vi "extract data to circle.vi"(5 "Circles (Shape Detection 1)":T1(array[cluster]) {"Position"."Y" format="%.2f"; "Position"."X" format="%.2f"}) -> (0 "Circles":cluster{"x":dbl, "y":dbl, "r":dbl}[](array[cluster]), 1 "y":dbl[](array[numeric]), 2 "x":dbl[](array[numeric]))   [LabVIEW 2018]
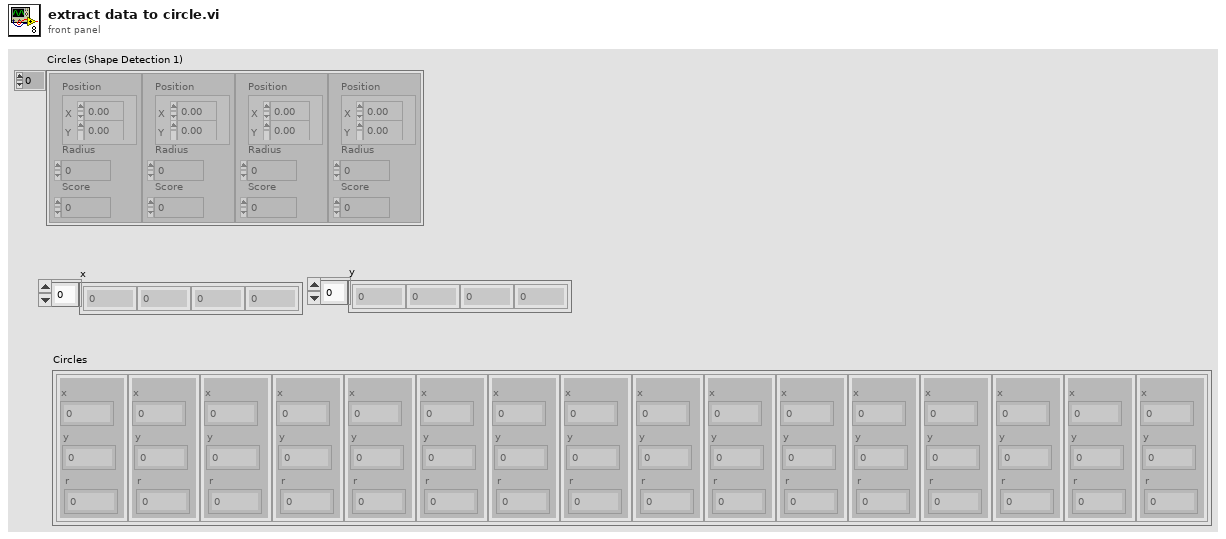
[diagram p1: front panel]
types:
  T1 = cluster{"Position":cluster{"X":sgl, "Y":sgl}, "Radius":dbl, "Score":dbl}[]
  T2 = cluster{"element":dbl, "element":dbl, "element":dbl}
  T3 = cluster{"element":dbl, "element":dbl, "element":dbl}[]
  T4 = cluster{"Position":cluster{"X":sgl, "Y":sgl}, "Radius":dbl, "Score":dbl}
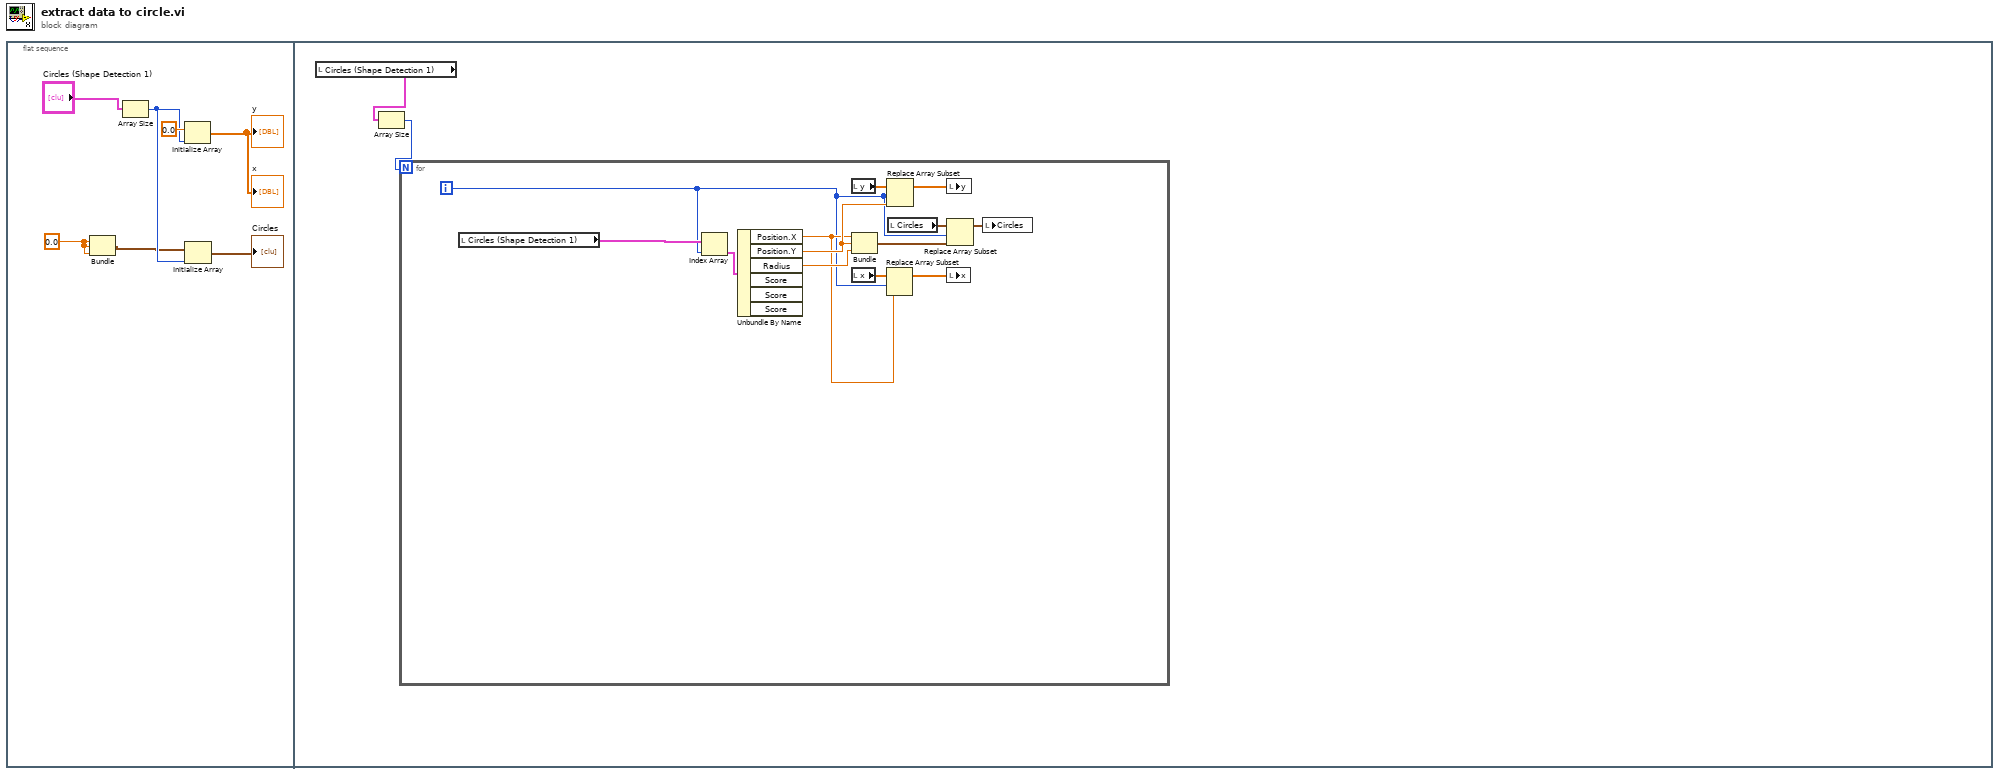
[diagram p0: block diagram]
diagram:
  n1 = flat-sequence {
    frame #0 {
      w1 = 0.0 ("element")
      n2 = Bundle("element"=w1, "element"=w1, "element"=w1) -> (w2:T2)  [unwired: 1 in]
      n3 = Array Size(array="Circles (Shape Detection 1)") -> (size(s)=w3:i32)
      n4 = Initialize Array(0.0 ("element"), w3) -> (→"x" →"y":dbl[])
      n5 = Initialize Array(w2, w3) -> (→"Circles":T3)
    }
    frame #1 {
      n6 = local read "Circles (Shape Detection 1)"() -> (w9:T1)
      n7 = Array Size(array=w9) -> (size(s)=w8:i32)
      n8 = for {
        N: w8 -> [_]
        i -> [w10]
        n9 = local read "Circles (Shape Detection 1)"() -> (w22:T1)
        n10 = Index Array(array=w22, index=w10) -> (element=w21:T4)
        n11 = Unbundle By Name(w21) -> ("Position.X"=w15:sgl, "Position.Y"=w16:sgl, "Radius"=w20:dbl)  [unwired: 3 out]
        n12 = local read "y"() -> (w12:dbl[])
        n13 = Bundle("X"=w15, "Y"=w16, "Radius"=w20) -> (w18:cluster{"X":sgl, "Y":sgl, "Radius":dbl})  [unwired: 1 in]
        n14 = local read "x"() -> (w14:dbl[])
        n15 = Replace Array Subset(array=w14, new element=w15, index=w10) -> (w13:dbl[])
        n16 = Replace Array Subset(array=w12, new element=w16, index=w10) -> (w11:dbl[])
        n17 = local read "Circles"() -> (w19:cluster{"x":dbl, "y":dbl, "r":dbl}[])
        n18 = local write "y"(w11) -> ()
        n19 = Replace Array Subset(array=w19, new element=w18, index=w10) -> (w17:cluster{"x":dbl, "y":dbl, "r":dbl}[])
        n20 = local write "x"(w13) -> ()
        n21 = local write "Circles"(w17) -> ()
      }
    }
  }
